vi "Autonomous Independent.vi"() -> ()   [LabVIEW 2016]
doc: "This VI is called when autonomous begins, and will automatically be terminated when autonomous ends. You can carry out timed or sensor driven robot movement independently without needing to return to the caller."
uses:
  <vilib>/Rock Robotics/WPI/Solenoid/WPI_SolenoidSetEnum.vi
  <vilib>/Rock Robotics/WPI/Utilities/WPI_GetSetVariantRefNum.vi
  <vilib>/Rock Robotics/WPI/RobotDrive/WPI_RobotDriveArcadeDrive_Standard(NoSaturation).vi
  <vilib>/Rock Robotics/Network Tables/NT Write Numeric Array.vi
  <vilib>/Rock Robotics/Network Tables/NT Read String.vi
panel:
  out "Current Movement, for debugging":T1 {"Y Joystick Value" scale=1.0..-1.0; "X Joystick Value" scale=-1.0..1.0}
  in  "Array of robot movements":T2(array[cluster])=[{"X Joystick Value"=0.39393939393939403, "Y Joystick Value"=0.0, "Delay (sec)"=1.0, "Movement Name"="turn"}, {"X Joystick Value"=-0.3737373737373737, "Y Joystick Value"=0.0, "Delay (sec)"=1.0, "Movement Name"="turn back"}] {"Y Joystick Value" scale=1.0..-1.0; "X Joystick Value" scale=-1.0..1.0}
  # "Be sure to right-click and choose Data Operations>>Make Current Value default if you want to save the array values with the VI"
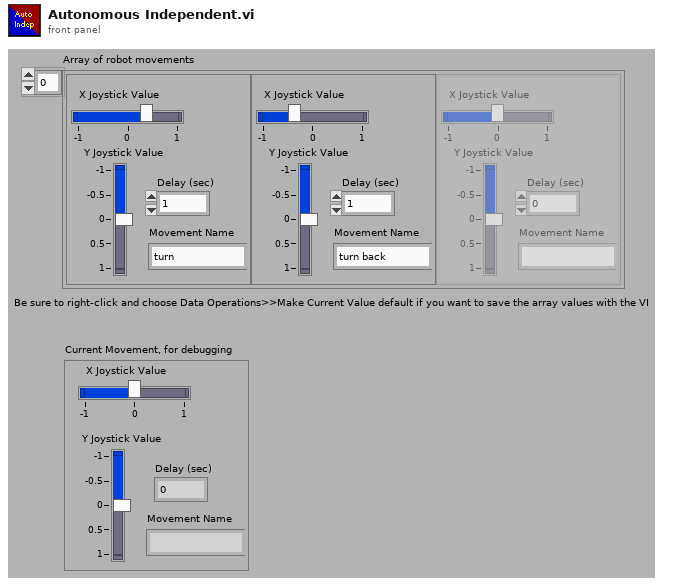
[diagram p1: front panel]
types:
  T1 = cluster{"X Joystick Value":dbl, "Y Joystick Value":dbl, "Delay (sec)":dbl, "Movement Name":string}
  T2 = cluster{"X Joystick Value":dbl, "Y Joystick Value":dbl, "Delay (sec)":dbl, "Movement Name":string}[]
  T3 = typedef "WPI_JoystickDevRef.ctl" = cluster{"Device":T4}
  T4 = typedef "WPI_JoystickDeviceEnum.ctl" = enum16{"USB 0", "USB 1", "USB 2", "USB 3", "USB 4", "USB 5"}
  T5 = typedef "WPI_RobotDriveDevRef.ctl" = cluster{"DevStatus":errorcluster, "Motors[]":T6[], "Square Inputs":bool, "Max Output":dbl}
  T6 = typedef "WPI_MotorControlDeviceRef.ctl" = cluster{"DeviceStatus":errorcluster, "Type":T7, "PWM":cluster{"PWM Channel":T8, "DeadBand":T9}, "CAN":cluster{"Device Number":u8, "SetOutput VI Ref":variant, "GetOutput VI Ref":variant, "Enable VI Ref":variant, "Disable VI Ref":variant, "Data":variant}, "Invert":bool}
  T7 = typedef "WPI_MotorControlType.ctl" = enum16{"PWM", "CAN"}
  T8 = typedef "FPGA_DIOPWMChannel.ctl" = enum8{"PWM 0", "PWM 1", "PWM 2", "PWM 3", "PWM 4", "PWM 5", "PWM 6", "PWM 7", "PWM 8", "PWM 9", "PWM MXP 0", "PWM MXP 1", "PWM MXP 2", "PWM MXP 3", "PWM MXP 4", "PWM MXP 5", "PWM MXP 6", "PWM MXP 7", "PWM MXP 8", "PWM MXP 9", "Invalid"}
  T9 = typedef "WPI_PWMDeadband.ctl" = cluster{"Name":string, "maxPositivePwm":i32, "minPositivePwm":i32, "centerPwm":i32, "maxNegativePwm":i32, "minNegativePwm":i32, "angularRange":u16}
  T10 = typedef "WPI_SolenoidDevRef.ctl" = cluster{"DevStatus":errorcluster, "Pneumatics Control Module":u8, "Forward Solenoid Channel":T11, "Reverse Solenoid Channel":T11}
  T11 = typedef "WPI_SolenoidChannel.ctl" = enum8{"Solenoid 0", "Solenoid 1", "Solenoid 2", "Solenoid 3", "Solenoid 4", "Solenoid 5", "Solenoid 6", "Solenoid 7", "Invalid"}
  T12 = typedef "WPI_SolenoidValue.ctl" = enum16{"Off", "On", "Forward", "Reverse"}
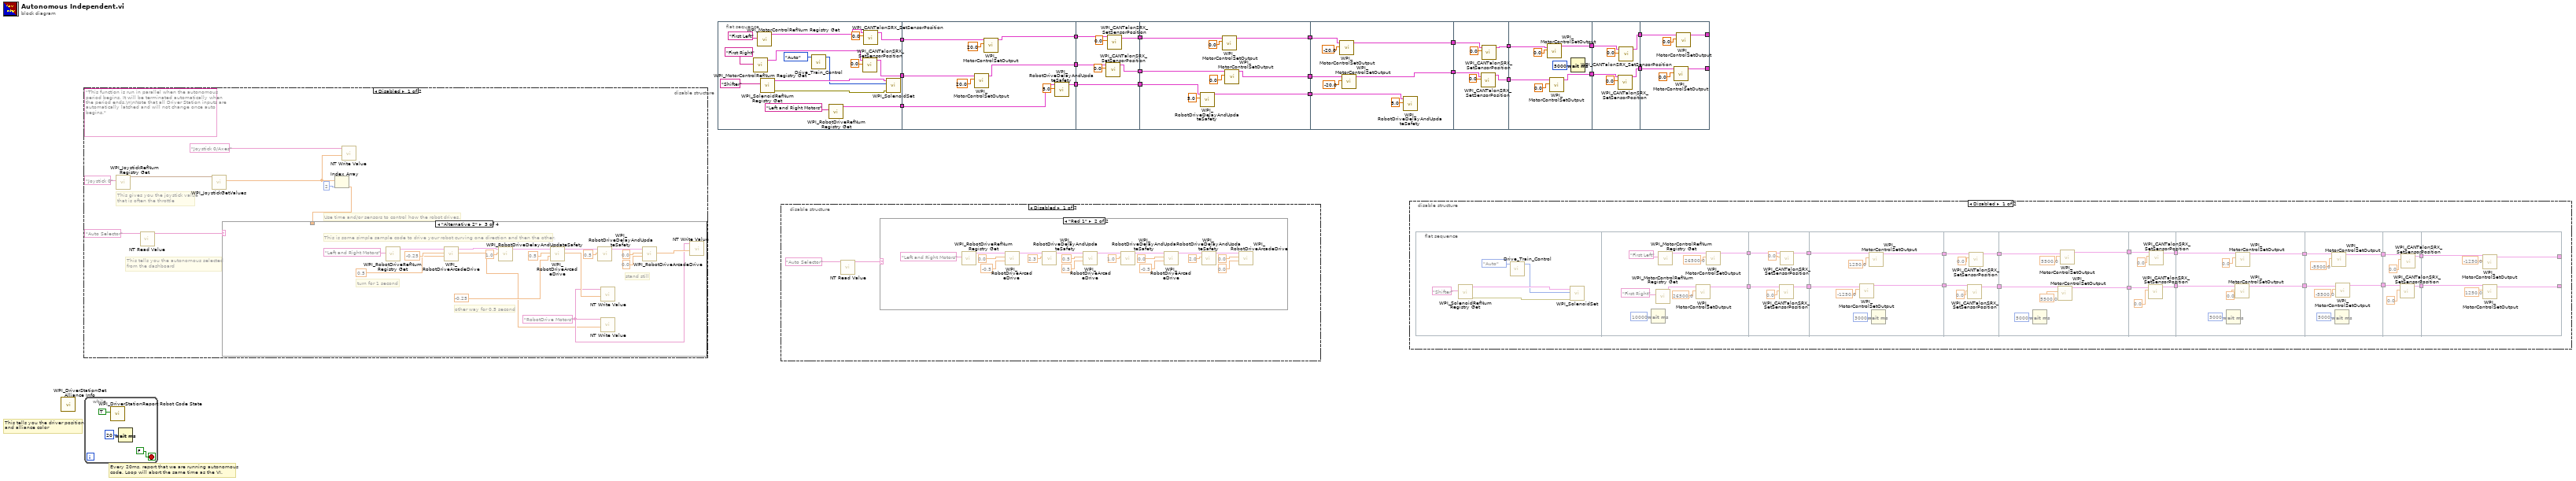
[diagram p0: block diagram]
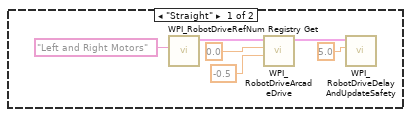
[diagram p3: hidden frame]
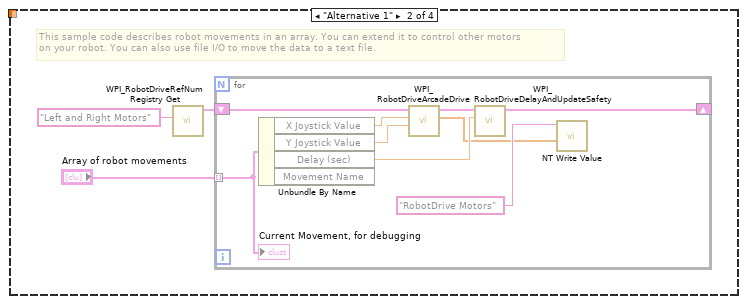
[diagram p6: hidden frame]
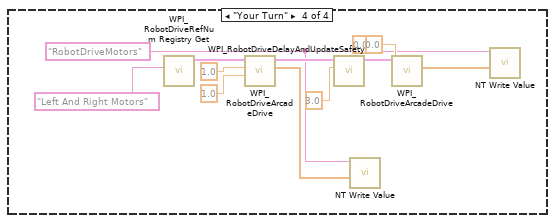
[diagram p7: hidden frame]
diagram:
  # "Every 20ms, report that we are running autonomous\ncode. Loop will abort the same time as the VI."
  # "This tells you the driver position\nand alliance color"
  n1 = call <vilib>:"WPI_DriverStationGet Alliance Info.vi"() -> ()  [unwired: 12 out]
  n2 = disable-structure shown="Disabled" {
    frame Disabled {
      (unwired) "This function is run in parallel when the autonomous period begins. It will be terminated automatically when the period ends.\n\nNote that all Driver Station inputs are automatically latched and will not change once auto begins."
      # "This tells you the autonomous selected\nfrom the dashboard"
      # "This gives you the joystick value\nthat is often the throttle"
      # "Use time and/or sensors to control how the robot drives."
      n3 = call <vilib>:"WPI_JoystickRefNum Registry Get.vi"("refnum name"="Joystick 0") -> ("JoystickDevRef"=w27:T3)  [unwired: 1 in, 9 out]
      n4 = call-poly <vilib>:"NT Read Value.vi"("Name"="Auto Selector") -> ("String"=w24:string)  [unwired: 9 in, 1 out]
      n5 = call <vilib>:"WPI_JoystickGetValues.vi"("JoystickDevRef"=w27) -> ("Axes"=w23:dbl[])  [unwired: 6 in, 4 out]
      n6 = Index Array(array=w23, index=2) -> (element=w21:dbl)
      n7 = case shown="\"Alternative 2\"" w24 {
        tunnel: w21 -> [_ _ _ _]
        frame Default {
          # "You can put your main auto here, or you can right-click on the case and make any\nother frame be the default case."
          # "This is the frame that will execute if no selection is made, or if it is not recognized"
        }
        frame "Alternative 1" {
          # "This sample code describes robot movements in an array. You can extend it to control other motors\non your robot. You can also use file I/O to move the data to a text file."
          n8 = call <vilib>:"WPI_RobotDriveRefNum Registry Get.vi"("refnum name"="Left and Right Motors") -> ("RobotDriveDevRef"=w30:T5)  [unwired: 1 in, 9 out]
          n9 = for {
            shift-right: [w38] -> _
            shift-left: w30 -> [w39]
            tunnel: "Array of robot movements" -> [w34] mode=indexing
            n10 = Unbundle By Name(w34) -> ("X Joystick Value"=w37:dbl, "Y Joystick Value"=w36:dbl, "Delay (sec)"=w35:dbl)  [unwired: 1 out]
            n11 = call-poly <vilib>:"WPI_RobotDriveArcadeDrive.vi"("Y axis value"=w36, "X axis value"=w37, "RobotDriveDevRef"=w39) -> ("Motor Values"=w32:dbl[], "RobotDriveDevRef"=w40:T5)  [unwired: 1 in, 6 out]
            n12 = call <vilib>:"WPI_RobotDriveDelayAndUpdateSafety.vi"("Delay (s)"=w35, "RobotDriveDevRef"=w40) -> ("RobotDriveDevRef 2"=w38:T5)  [unwired: 8 in, 1 out]
            n13 = call-poly <vilib>:"NT Write Value.vi"("Numeric Array"=w32, "Name"="RobotDrive Motors") -> ()  [unwired: 9 in, 1 out]
            "Current Movement, for debugging" <- w34
          }
        }
        frame "Alternative 2" {
          w42 = "RobotDrive Motors" ("Name")
          # "This is some simple sample code to drive your robot curving one direction and then the other."
          # "stand still"
          # "other way for 0.5 second"
          # "turn for 1 second"
          n14 = call <vilib>:"WPI_RobotDriveRefNum Registry Get.vi"("refnum name"="Left and Right Motors") -> ("RobotDriveDevRef"=w58:T5)  [unwired: 1 in, 9 out]
          n15 = call-poly <vilib>:"WPI_RobotDriveArcadeDrive.vi"("Y axis value"=0.5 ("X axis value"), "X axis value"=-0.25, "RobotDriveDevRef"=w58) -> ("Motor Values"=w41:dbl[], "RobotDriveDevRef"=w51:T5)  [unwired: 1 in, 6 out]
          n16 = call <vilib>:"WPI_RobotDriveDelayAndUpdateSafety.vi"("Delay (s)"=1.0, "RobotDriveDevRef"=w51) -> ("RobotDriveDevRef 2"=w52:T5)  [unwired: 8 in, 1 out]
          n17 = call-poly <vilib>:"WPI_RobotDriveArcadeDrive.vi"("Y axis value"=-0.25 ("X axis value"), "X axis value"=0.5, "RobotDriveDevRef"=w52) -> ("Motor Values"=w43:dbl[], "RobotDriveDevRef"=w53:T5)  [unwired: 1 in, 6 out]
          n18 = call <vilib>:"WPI_RobotDriveDelayAndUpdateSafety.vi"("Delay (s)"=0.5, "RobotDriveDevRef"=w53) -> ("RobotDriveDevRef 2"=w54:T5)  [unwired: 8 in, 1 out]
          n19 = call-poly <vilib>:"NT Write Value.vi"("Numeric Array"=w43, "Name"=w42) -> ()  [unwired: 9 in, 1 out]
          n20 = call-poly <vilib>:"NT Write Value.vi"("Numeric Array"=w41, "Name"=w42) -> ()  [unwired: 9 in, 1 out]
          n21 = call-poly <vilib>:"WPI_RobotDriveArcadeDrive.vi"("Y axis value"=0.0 ("X axis value"), "X axis value"=0.0, "RobotDriveDevRef"=w54) -> ("Motor Values"=w44:dbl[])  [unwired: 1 in, 7 out]
          n22 = call-poly <vilib>:"NT Write Value.vi"("Numeric Array"=w44, "Name"=w42) -> ()  [unwired: 9 in, 1 out]
        }
        frame "Your Turn" {
          w60 = "RobotDriveMotors" ("Name")
          n23 = call <vilib>:"WPI_RobotDriveRefNum Registry Get.vi"("refnum name"="Left And Right Motors") -> ("RobotDriveDevRef"=w64:T5)  [unwired: 1 in, 9 out]
          n24 = call-poly <vilib>:"WPI_RobotDriveArcadeDrive.vi"("Y axis value"=1.0, "X axis value"=1.0, "RobotDriveDevRef"=w64) -> ("Motor Values"=w70:dbl[], "RobotDriveDevRef"=w69:T5)  [unwired: 1 in, 6 out]
          n25 = call <vilib>:"WPI_RobotDriveDelayAndUpdateSafety.vi"("Delay (s)"=3.0 ("Feed time (s)"), "RobotDriveDevRef"=w69) -> ("RobotDriveDevRef 2"=w66:T5)  [unwired: 8 in, 1 out]
          n26 = call-poly <vilib>:"NT Write Value.vi"("Numeric Array"=w70, "Name"=w60) -> ()  [unwired: 9 in, 1 out]
          n27 = call-poly <vilib>:"WPI_RobotDriveArcadeDrive.vi"("Y axis value"=0.0, "X axis value"=0.0, "RobotDriveDevRef"=w66) -> ("Motor Values"=w65:dbl[])  [unwired: 1 in, 7 out]
          n28 = call-poly <vilib>:"NT Write Value.vi"("Numeric Array"=w65, "Name"=w60) -> ()  [unwired: 9 in, 1 out]
        }
      }
      n29 = call-poly <vilib>:"NT Write Value.vi"("Numeric Array"=w23, "Name"="Joystick 0/Axes") -> ()  [unwired: 9 in, 1 out]
    }
    frame Enabled {
    }
  }
  n30 = while {
    stop <- FALSE stop-if-true
    n31 = call <vilib>:"WPI_DriverStationReport Robot Code State.vi"("Autonomous"=TRUE) -> ()  [unwired: 10 in, 1 out]
    n32 = Wait (ms)(milliseconds to wait=u32 20) -> ()  [unwired: 1 out]
  }
  n33 = flat-sequence {
    tunnel: [w78] -> w6
    tunnel: [w76] -> w5
    tunnel: [w74] -> w4
    tunnel: [w95] -> w20
    tunnel: [w94] -> w19
    tunnel: w6 -> [w93]
    tunnel: w5 -> [w92]
    tunnel: w4 -> [w91]
    tunnel: [w89] -> w2
    tunnel: w20 -> [w104]
    tunnel: w19 -> [w103]
    tunnel: [w102] -> w18
    tunnel: [w101] -> w17
    tunnel: [w98] -> w3
    tunnel: w2 -> [w98]
    tunnel: w18 -> [w111]
    tunnel: w17 -> [w110]
    tunnel: [w109] -> w16
    tunnel: [w108] -> w15
    tunnel: w3 -> [w106]
    tunnel: [w105] -> w1
    tunnel: w16 -> [w119]
    tunnel: w15 -> [w118]
    tunnel: [w117] -> w14
    tunnel: [w116] -> w13
    tunnel: w1 -> [w114]
    tunnel: w14 -> [w125]
    tunnel: w13 -> [w124]
    tunnel: [w123] -> w12
    tunnel: [w122] -> w11
    tunnel: w12 -> [w132]
    tunnel: w11 -> [w131]
    tunnel: [w130] -> w10
    tunnel: [w129] -> w9
    tunnel: w10 -> [w138]
    tunnel: w9 -> [w137]
    tunnel: [w136] -> w8
    tunnel: [w135] -> w7
    tunnel: w8 -> [w144]
    tunnel: w7 -> [w143]
    tunnel: [w142] -> _
    tunnel: [w141] -> _
    frame #0 {
      n34 = call <vilib>:"WPI_MotorControlRefNum Registry Get.vi"("refnum name"="First Right") -> ("MotorControlDevRef"=w79:T6)  [unwired: 9 in, 1 out]
      n35 = call <vilib>:"WPI_MotorControlRefNum Registry Get.vi"("refnum name"="First Left") -> ("MotorControlDevRef"=w77:T6)  [unwired: 9 in, 1 out]
      n36 = call <vilib>:"WPI_SolenoidRefNum Registry Get.vi"("refnum name"="Shifter") -> ("error out"=w85:errorcluster, "SolenoidDevRef"=w86:T10)  [unwired: 9 in]
      n37 = call "Drive_Train_Control.vi"("Command"=enum16{"Run", "Init", "Auto"}."Auto") -> ("Value"=w84:T12)  [unwired: 10 in]
      n38 = call <vilib>:"WPI_RobotDriveRefNum Registry Get.vi"("refnum name"="Left and Right Motors") -> ("RobotDriveDevRef"=w74:T5)  [unwired: 1 in, 9 out]
      n39 = call <vilib>:"WPI_CANTalonSRX_SetSensorPosition.vi"("New Sensor Position"=0.0, "CAN Talon SRX Ref"=w79) -> ("CAN Talon SRX Ref"=w78:T6)  [unwired: 8 in, 1 out]
      n40 = call <vilib>:"WPI_CANTalonSRX_SetSensorPosition.vi"("New Sensor Position"=0.0, "CAN Talon SRX Ref"=w77) -> ("CAN Talon SRX Ref"=w76:T6)  [unwired: 8 in, 1 out]
      n41 = call-poly <vilib>:"WPI_SolenoidSet.vi"("error in (no error)"=w85, "Value"=w84, "SolenoidDevRef"=w86) -> ()  [unwired: 7 in, 2 out]
    }
    frame #1 {
      n42 = call <vilib>:"WPI_MotorControlSetOutput.vi"("Output"=20.0, "MotorControlDevRef"=w93) -> ("MotorControlDevRef"=w94:T6)  [unwired: 7 in, 2 out]
      n43 = call <vilib>:"WPI_MotorControlSetOutput.vi"("Output"=20.0, "MotorControlDevRef"=w92) -> ("MotorControlDevRef"=w95:T6)  [unwired: 7 in, 2 out]
      n44 = call <vilib>:"WPI_RobotDriveDelayAndUpdateSafety.vi"("Delay (s)"=5.0, "RobotDriveDevRef"=w91) -> ("RobotDriveDevRef 2"=w89:T5)  [unwired: 8 in, 1 out]
    }
    frame #2 {
      n45 = call <vilib>:"WPI_CANTalonSRX_SetSensorPosition.vi"("New Sensor Position"=0.0, "CAN Talon SRX Ref"=w103) -> ("CAN Talon SRX Ref"=w102:T6)  [unwired: 8 in, 1 out]
      n46 = call <vilib>:"WPI_CANTalonSRX_SetSensorPosition.vi"("New Sensor Position"=0.0, "CAN Talon SRX Ref"=w104) -> ("CAN Talon SRX Ref"=w101:T6)  [unwired: 8 in, 1 out]
    }
    frame #3 {
      n47 = call <vilib>:"WPI_RobotDriveDelayAndUpdateSafety.vi"("Delay (s)"=5.0, "RobotDriveDevRef"=w106) -> ("RobotDriveDevRef 2"=w105:T5)  [unwired: 8 in, 1 out]
      n48 = call <vilib>:"WPI_MotorControlSetOutput.vi"("Output"=0.0, "MotorControlDevRef"=w110) -> ("MotorControlDevRef"=w109:T6)  [unwired: 7 in, 2 out]
      n49 = call <vilib>:"WPI_MotorControlSetOutput.vi"("Output"=0.0, "MotorControlDevRef"=w111) -> ("MotorControlDevRef"=w108:T6)  [unwired: 7 in, 2 out]
    }
    frame #4 {
      n50 = call <vilib>:"WPI_MotorControlSetOutput.vi"("Output"=-20.0, "MotorControlDevRef"=w119) -> ("MotorControlDevRef"=w117:T6)  [unwired: 7 in, 2 out]
      n51 = call <vilib>:"WPI_MotorControlSetOutput.vi"("Output"=-20.0, "MotorControlDevRef"=w118) -> ("MotorControlDevRef"=w116:T6)  [unwired: 7 in, 2 out]
      n52 = call <vilib>:"WPI_RobotDriveDelayAndUpdateSafety.vi"("Delay (s)"=5.0, "RobotDriveDevRef"=w114) -> ()  [unwired: 8 in, 2 out]
    }
    frame #5 {
      n53 = call <vilib>:"WPI_CANTalonSRX_SetSensorPosition.vi"("New Sensor Position"=0.0, "CAN Talon SRX Ref"=w124) -> ("CAN Talon SRX Ref"=w122:T6)  [unwired: 8 in, 1 out]
      n54 = call <vilib>:"WPI_CANTalonSRX_SetSensorPosition.vi"("New Sensor Position"=0.0, "CAN Talon SRX Ref"=w125) -> ("CAN Talon SRX Ref"=w123:T6)  [unwired: 8 in, 1 out]
    }
    frame #6 {
      n55 = call <vilib>:"WPI_MotorControlSetOutput.vi"("Output"=0.0, "MotorControlDevRef"=w132) -> ("MotorControlDevRef"=w130:T6)  [unwired: 7 in, 2 out]
      n56 = call <vilib>:"WPI_MotorControlSetOutput.vi"("Output"=0.0, "MotorControlDevRef"=w131) -> ("MotorControlDevRef"=w129:T6)  [unwired: 7 in, 2 out]
      n57 = Wait (ms)(milliseconds to wait=u32 5000) -> ()  [unwired: 1 out]
    }
    frame #7 {
      n58 = call <vilib>:"WPI_CANTalonSRX_SetSensorPosition.vi"("New Sensor Position"=0.0, "CAN Talon SRX Ref"=w137) -> ("CAN Talon SRX Ref"=w135:T6)  [unwired: 8 in, 1 out]
      n59 = call <vilib>:"WPI_CANTalonSRX_SetSensorPosition.vi"("New Sensor Position"=0.0, "CAN Talon SRX Ref"=w138) -> ("CAN Talon SRX Ref"=w136:T6)  [unwired: 8 in, 1 out]
    }
    frame #8 {
      n60 = call <vilib>:"WPI_MotorControlSetOutput.vi"("Output"=0.0, "MotorControlDevRef"=w143) -> ("MotorControlDevRef"=w141:T6)  [unwired: 7 in, 2 out]
      n61 = call <vilib>:"WPI_MotorControlSetOutput.vi"("Output"=0.0, "MotorControlDevRef"=w144) -> ("MotorControlDevRef"=w142:T6)  [unwired: 7 in, 2 out]
    }
  }
  n62 = disable-structure shown="Disabled" {
    frame Disabled {
      n63 = call-poly <vilib>:"NT Read Value.vi"("Name"="Auto Selector") -> ("String"=w148:string)  [unwired: 9 in, 1 out]
      n64 = case shown="\"Red 1\"" w148 {
        frame "Straight" {
          n65 = call <vilib>:"WPI_RobotDriveRefNum Registry Get.vi"("refnum name"="Left and Right Motors") -> ("RobotDriveDevRef"=w154:T5)  [unwired: 1 in, 9 out]
          n66 = call-poly <vilib>:"WPI_RobotDriveArcadeDrive.vi"("Y axis value"=-0.5, "X axis value"=0.0, "RobotDriveDevRef"=w154) -> ("RobotDriveDevRef"=w151:T5)  [unwired: 1 in, 7 out]
          n67 = call <vilib>:"WPI_RobotDriveDelayAndUpdateSafety.vi"("Delay (s)"=5.0, "RobotDriveDevRef"=w151) -> ()  [unwired: 8 in, 2 out]
        }
        frame "Red 1" {
          n68 = call <vilib>:"WPI_RobotDriveRefNum Registry Get.vi"("refnum name"="Left and Right Motors") -> ("RobotDriveDevRef"=w157:T5)  [unwired: 1 in, 9 out]
          n69 = call-poly <vilib>:"WPI_RobotDriveArcadeDrive.vi"("Y axis value"=-0.5, "X axis value"=0.0, "RobotDriveDevRef"=w157) -> ("RobotDriveDevRef"=w160:T5)  [unwired: 1 in, 7 out]
          n70 = call <vilib>:"WPI_RobotDriveDelayAndUpdateSafety.vi"("Delay (s)"=2.3, "RobotDriveDevRef"=w160) -> ("RobotDriveDevRef 2"=w156:T5)  [unwired: 8 in, 1 out]
          n71 = call-poly <vilib>:"WPI_RobotDriveArcadeDrive.vi"("Y axis value"=0.5, "X axis value"=0.5, "RobotDriveDevRef"=w156) -> ("RobotDriveDevRef"=w164:T5)  [unwired: 1 in, 7 out]
          n72 = call <vilib>:"WPI_RobotDriveDelayAndUpdateSafety.vi"("Delay (s)"=1.0, "RobotDriveDevRef"=w164) -> ("RobotDriveDevRef 2"=w155:T5)  [unwired: 8 in, 1 out]
          n73 = call-poly <vilib>:"WPI_RobotDriveArcadeDrive.vi"("Y axis value"=-0.5, "X axis value"=0.0, "RobotDriveDevRef"=w155) -> ("RobotDriveDevRef"=w168:T5)  [unwired: 1 in, 7 out]
          n74 = call <vilib>:"WPI_RobotDriveDelayAndUpdateSafety.vi"("Delay (s)"=2.0, "RobotDriveDevRef"=w168) -> ("RobotDriveDevRef 2"=w171:T5)  [unwired: 8 in, 1 out]
          n75 = call-poly <vilib>:"WPI_RobotDriveArcadeDrive.vi"("Y axis value"=0.0, "X axis value"=0.0, "RobotDriveDevRef"=w171) -> ()  [unwired: 1 in, 8 out]
        }
      }
    }
    frame Enabled {
    }
  }
  n76 = disable-structure shown="Disabled" {
    frame Disabled {
      n77 = flat-sequence {
        tunnel: [w198] -> w191
        tunnel: [w197] -> w190
        tunnel: w191 -> [w209]
        tunnel: [w208] -> w189
        tunnel: [w207] -> w188
        tunnel: w190 -> [w206]
        tunnel: w189 -> [w216]
        tunnel: [w215] -> w187
        tunnel: w188 -> [w214]
        tunnel: [w213] -> w186
        tunnel: [w222] -> w185
        tunnel: w187 -> [w221]
        tunnel: [w220] -> w184
        tunnel: w186 -> [w219]
        tunnel: w185 -> [w229]
        tunnel: w184 -> [w228]
        tunnel: [w227] -> w183
        tunnel: [w226] -> w182
        tunnel: w183 -> [w235]
        tunnel: w182 -> [w234]
        tunnel: [w233] -> w181
        tunnel: [w232] -> w180
        tunnel: [w243] -> w179
        tunnel: w181 -> [w242]
        tunnel: w180 -> [w241]
        tunnel: [w240] -> w178
        tunnel: w179 -> [w250]
        tunnel: w178 -> [w249]
        tunnel: [w248] -> w177
        tunnel: [w247] -> w176
        tunnel: w177 -> [w255]
        tunnel: w176 -> [w254]
        tunnel: [w253] -> w175
        tunnel: [w252] -> w174
        tunnel: w175 -> [w262]
        tunnel: w174 -> [w261]
        tunnel: [w259] -> _
        tunnel: [w258] -> _
        frame #0 {
          n78 = call <vilib>:"WPI_SolenoidRefNum Registry Get.vi"("refnum name"="Shifter") -> ("error out"=w193:errorcluster, "SolenoidDevRef"=w194:T10)  [unwired: 9 in]
          n79 = call "Drive_Train_Control.vi"("Command"=enum16{"Run", "Init", "Auto"}."Auto") -> ("Value"=w192:T12)  [unwired: 10 in]
          n80 = call-poly <vilib>:"WPI_SolenoidSet.vi"("error in (no error)"=w193, "Value"=w192, "SolenoidDevRef"=w194) -> ()  [unwired: 7 in, 2 out]
        }
        frame #1 {
          n81 = Wait (ms)(milliseconds to wait=u32 10000) -> ()  [unwired: 1 out]
          n82 = call <vilib>:"WPI_MotorControlRefNum Registry Get.vi"("refnum name"="First Right") -> ("MotorControlDevRef"=w201:T6)  [unwired: 9 in, 1 out]
          n83 = call <vilib>:"WPI_MotorControlRefNum Registry Get.vi"("refnum name"="First Left") -> ("MotorControlDevRef"=w203:T6)  [unwired: 9 in, 1 out]
          n84 = call <vilib>:"WPI_MotorControlSetOutput.vi"("Output"=26500.0, "MotorControlDevRef"=w201) -> ("MotorControlDevRef"=w197:T6)  [unwired: 7 in, 2 out]
          n85 = call <vilib>:"WPI_MotorControlSetOutput.vi"("Output"=26500.0, "MotorControlDevRef"=w203) -> ("MotorControlDevRef"=w198:T6)  [unwired: 7 in, 2 out]
        }
        frame #2 {
          n86 = call <vilib>:"WPI_CANTalonSRX_SetSensorPosition.vi"("New Sensor Position"=0.0, "CAN Talon SRX Ref"=w206) -> ("CAN Talon SRX Ref"=w208:T6)  [unwired: 8 in, 1 out]
          n87 = call <vilib>:"WPI_CANTalonSRX_SetSensorPosition.vi"("New Sensor Position"=0.0, "CAN Talon SRX Ref"=w209) -> ("CAN Talon SRX Ref"=w207:T6)  [unwired: 8 in, 1 out]
        }
        frame #3 {
          n88 = call <vilib>:"WPI_MotorControlSetOutput.vi"("Output"=-1250.0, "MotorControlDevRef"=w216) -> ("MotorControlDevRef"=w215:T6)  [unwired: 7 in, 2 out]
          n89 = call <vilib>:"WPI_MotorControlSetOutput.vi"("Output"=1250.0, "MotorControlDevRef"=w214) -> ("MotorControlDevRef"=w213:T6)  [unwired: 7 in, 2 out]
          n90 = Wait (ms)(milliseconds to wait=u32 3000) -> ()  [unwired: 1 out]
        }
        frame #4 {
          n91 = call <vilib>:"WPI_CANTalonSRX_SetSensorPosition.vi"("New Sensor Position"=0.0, "CAN Talon SRX Ref"=w221) -> ("CAN Talon SRX Ref"=w220:T6)  [unwired: 8 in, 1 out]
          n92 = call <vilib>:"WPI_CANTalonSRX_SetSensorPosition.vi"("New Sensor Position"=0.0, "CAN Talon SRX Ref"=w219) -> ("CAN Talon SRX Ref"=w222:T6)  [unwired: 8 in, 1 out]
        }
        frame #5 {
          n93 = Wait (ms)(milliseconds to wait=u32 5000) -> ()  [unwired: 1 out]
          n94 = call <vilib>:"WPI_MotorControlSetOutput.vi"("Output"=5500.0, "MotorControlDevRef"=w228) -> ("MotorControlDevRef"=w226:T6)  [unwired: 7 in, 2 out]
          n95 = call <vilib>:"WPI_MotorControlSetOutput.vi"("Output"=5500.0, "MotorControlDevRef"=w229) -> ("MotorControlDevRef"=w227:T6)  [unwired: 7 in, 2 out]
        }
        frame #6 {
          n96 = call <vilib>:"WPI_CANTalonSRX_SetSensorPosition.vi"("New Sensor Position"=0.0, "CAN Talon SRX Ref"=w234) -> ("CAN Talon SRX Ref"=w232:T6)  [unwired: 8 in, 1 out]
          n97 = call <vilib>:"WPI_CANTalonSRX_SetSensorPosition.vi"("New Sensor Position"=0.0, "CAN Talon SRX Ref"=w235) -> ("CAN Talon SRX Ref"=w233:T6)  [unwired: 8 in, 1 out]
        }
        frame #7 {
          n98 = Wait (ms)(milliseconds to wait=u32 5000) -> ()  [unwired: 1 out]
          n99 = call <vilib>:"WPI_MotorControlSetOutput.vi"("Output"=0.0, "MotorControlDevRef"=w241) -> ("MotorControlDevRef"=w240:T6)  [unwired: 7 in, 2 out]
          n100 = call <vilib>:"WPI_MotorControlSetOutput.vi"("Output"=0.0, "MotorControlDevRef"=w242) -> ("MotorControlDevRef"=w243:T6)  [unwired: 7 in, 2 out]
        }
        frame #8 {
          n101 = call <vilib>:"WPI_MotorControlSetOutput.vi"("Output"=-5500.0, "MotorControlDevRef"=w250) -> ("MotorControlDevRef"=w247:T6)  [unwired: 7 in, 2 out]
          n102 = Wait (ms)(milliseconds to wait=u32 5000) -> ()  [unwired: 1 out]
          n103 = call <vilib>:"WPI_MotorControlSetOutput.vi"("Output"=-5500.0, "MotorControlDevRef"=w249) -> ("MotorControlDevRef"=w248:T6)  [unwired: 7 in, 2 out]
        }
        frame #9 {
          n104 = call <vilib>:"WPI_CANTalonSRX_SetSensorPosition.vi"("New Sensor Position"=0.0, "CAN Talon SRX Ref"=w255) -> ("CAN Talon SRX Ref"=w252:T6)  [unwired: 8 in, 1 out]
          n105 = call <vilib>:"WPI_CANTalonSRX_SetSensorPosition.vi"("New Sensor Position"=0.0, "CAN Talon SRX Ref"=w254) -> ("CAN Talon SRX Ref"=w253:T6)  [unwired: 8 in, 1 out]
        }
        frame #10 {
          n106 = call <vilib>:"WPI_MotorControlSetOutput.vi"("Output"=-1250.0, "MotorControlDevRef"=w262) -> ("MotorControlDevRef"=w259:T6)  [unwired: 7 in, 2 out]
          n107 = call <vilib>:"WPI_MotorControlSetOutput.vi"("Output"=1250.0, "MotorControlDevRef"=w261) -> ("MotorControlDevRef"=w258:T6)  [unwired: 7 in, 2 out]
        }
      }
    }
    frame Enabled {
    }
  }
